vi "ResampleWaveforms.vi"(9 "Numeric":dbl=0.0001 format="%#_13g", 10 "Waveform 2":waveform(dbl), 11 "Waveform":waveform(dbl)) -> (2 "resampled waveform out 2":waveform(dbl), 3 "resampled waveform out":waveform(dbl))   [LabVIEW 2023]
uses:
  <vilib>/measure/NI_MAPro.lvlib
  <vilib>/measure/maresamp.llb/Resample Waveform (single shot).vi
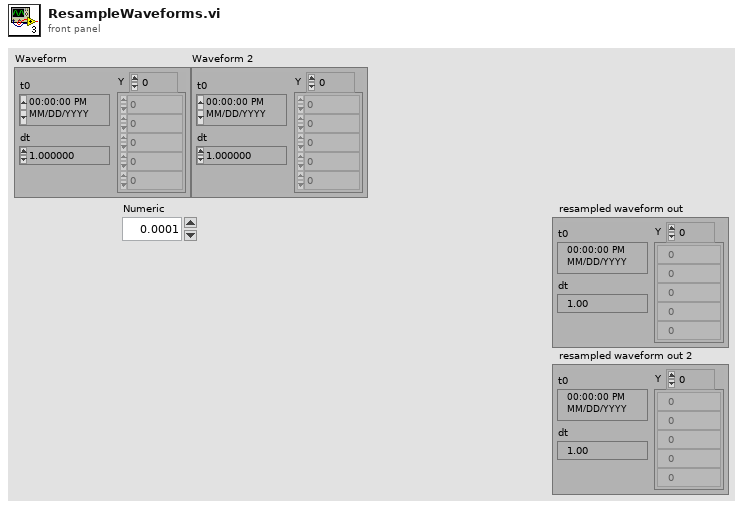
[diagram p1: front panel]
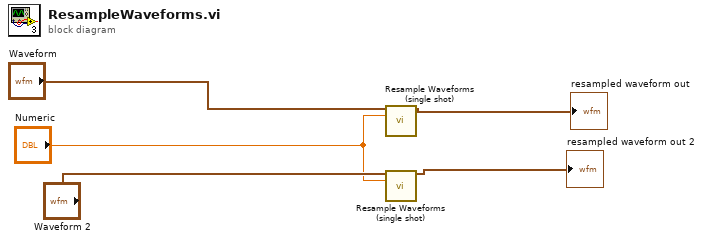
[diagram p0: block diagram]
diagram:
  n1 = call-poly <vilib>:"Resample Waveforms (single shot).vi"("waveform in"="Waveform", "dt"="Numeric") -> ("resampled waveform out"=→"resampled waveform out":waveform(dbl))  [unwired: 10 in, 3 out]
  n2 = call-poly <vilib>:"Resample Waveforms (single shot).vi"("waveform in"="Waveform 2", "dt"="Numeric") -> ("resampled waveform out"=→"resampled waveform out 2":waveform(dbl))  [unwired: 10 in, 3 out]
